vi "test-nisastevent.vi"() -> ()   [LabVIEW 2013]
uses:
  <resource>/importtools/Common/Event/NISAST Event.lvclass
panel:
  in  "确定按钮":bool
  out "Name":string
  in  "停止按钮":bool
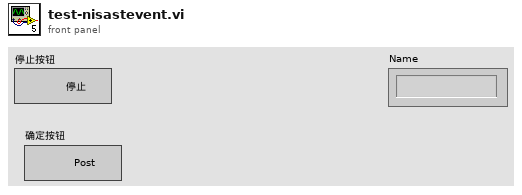
[diagram p1: front panel]
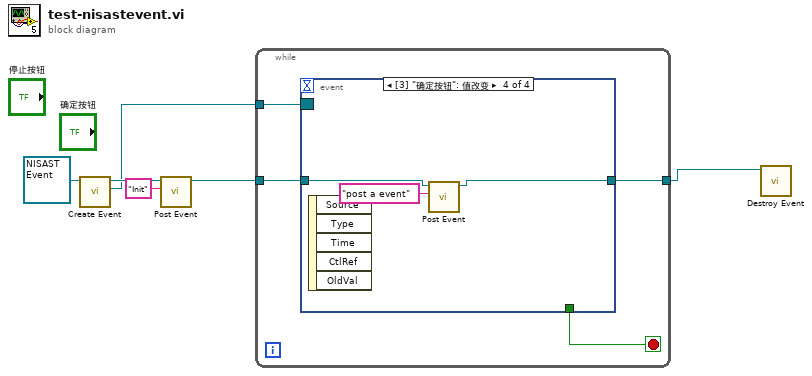
[diagram p0: block diagram]
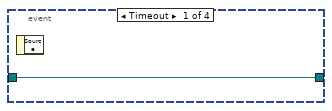
[diagram p2: hidden frame]
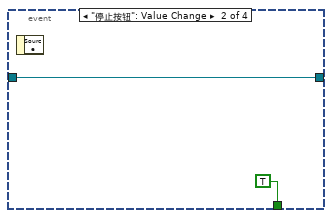
[diagram p3: hidden frame]
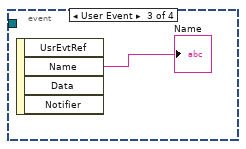
[diagram p4: hidden frame]
diagram:
  n1 = call-dynamic "Create Event.vi"("Event in"=refnum<class "NISAST Event.lvclass"> refnum) -> ("Event Registration Refnum"=w2:refnum<event-registration>, "Event out"=w5:refnum<class "NISAST Event.lvclass">)  [unwired: 8 in, 1 out]
  n2 = call-dynamic "Post Event.vi"("Event Name"="Init", "Event in"=w5) -> ("Event out"=w3:refnum<class "NISAST Event.lvclass">)  [unwired: 8 in, 1 out]
  n3 = while {
    tunnel: w3 -> [w8]
    tunnel: w2 -> [w10]
    tunnel: [w7] -> w1
    stop <- w9 stop-if-true
    n4 = event shown="[3] \"确定按钮\": 值改变" {
      selector: w10 -> [_ _ _ _]
      dyn-events: _ -> [_ _ _ _]
      timeout: _ -> [_ _ _ _]
      tunnel: [_ TRUE _ _] -> w9
      tunnel: w8 -> [w11 w12 _ w17]
      tunnel: [w11 w12 _ w16] -> w7
      event Timeout {
        n5 = event-data() -> ()  [unwired: 1 in, 1 out]
      }
      event "停止按钮": Value Change {
        n6 = event-data() -> ()  [unwired: 1 in, 1 out]
      }
      event User Event {
        n7 = event-data() -> ("Name"=→"Name":string)  [unwired: 1 in, 3 out]
      }
      event "确定按钮": Value Change {
        n8 = event-data() -> ()  [unwired: 1 in, 5 out]
        n9 = call-dynamic "Post Event.vi"("Event Name"="post a event", "Event in"=w17) -> ("Event out"=w16:refnum<class "NISAST Event.lvclass">)  [unwired: 8 in, 1 out]
      }
    }
  }
  n10 = call-dynamic "Destroy Event.vi"("Event in"=w1) -> ()  [unwired: 9 in, 2 out]
